vi "Set Simulator.vi"(7 "Module Name":string, 8 "error in (no error)":errorcluster, 9 "Acceleration":dbl, 10 "Velocity":dbl) -> (0 "error out":errorcluster)   [LabVIEW 2019, in "ADLINK Motion Card.lvlib"]
uses:
  ADLINK Motion Card.lvlib
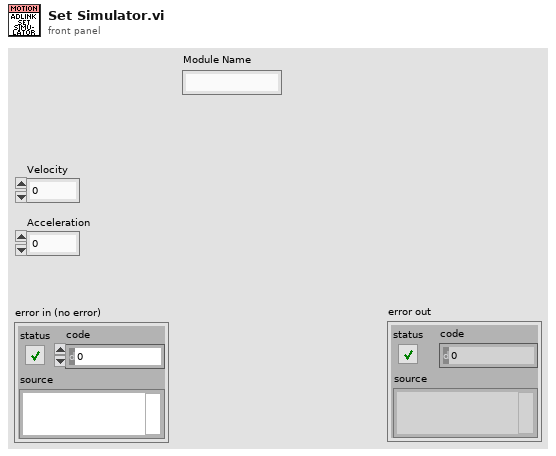
[diagram p1: front panel]
types:
  T1 = typedef "ADLINK Motion Card.lvlib/SEQ Data.ctl" = cluster{"Current Position":dbl, "Target Position":dbl, "Velocity":dbl, "Acceleration":dbl, "Arrived?":bool, "data value reference":refnum<data-value>, "VI Refnum":refnum<vi>}
  T2 = cluster{"Current Position":dbl, "Target Position":dbl, "Velocity":dbl, "Acceleration":dbl, "Arrived?":bool}
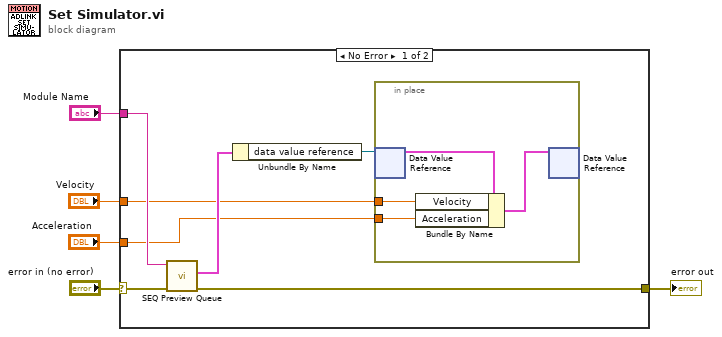
[diagram p0: block diagram]
diagram:
  n1 = case shown="No Error" "error in (no error)" {
    selector: "error in (no error)" -> [w11 w17]
    tunnel: [w6 w17] -> w5
    tunnel: "Module Name" -> [w12 _]
    tunnel: "Velocity" -> [w8 _]
    tunnel: "Acceleration" -> [w7 _]
    frame No Error {
      n2 = call "SEQ Preview Queue.vi"("error in (no error)"=w11, "Queue Name"=w12) -> ("error out"=w6:errorcluster, "Setting"=w10:T1)  [unwired: 8 in]
      n3 = Unbundle By Name(w10) -> ("data value reference"=w9:refnum<data-value>)
      n4 = in-place {
        in-place-border: w8 -> [w15]
        in-place-border: w7 -> [w14]
        n5 = in-place-dvr #1(w9) -> (w16:T2)  [unwired: 1 out]
        n6 = Bundle By Name(cluster=w16, "Velocity"=w15, "Acceleration"=w14) -> (w13:T2)
        n7 = in-place-dvr #1(w13) -> ()  [unwired: 2 out]
      }
    }
    frame Error {
    }
  }
  "error out" <- w5
